vi "Zernike_to_Mirror_Mode_Converter_v01.vi"(2 "Zernike Mode Amplitude":dbl, 3 "Zernike Mode":i32) -> (0 "Mirror Mode Amplitude":dbl[](array[numeric]), 1 "Mirror Modes":i32[](array[numeric]))   [LabVIEW 2015]
uses:
  <vilib>/Utility/file.llb/Read Delimited Spreadsheet (DBL).vi
panel:
  in  "Mirror to Zernike Mode Conversion":path=path "C:/Users/Mlodzianoski/Desktop/Microscope 2 Labview Programs/VIs/DM/MirrorMode_conversion_to_ZernikeMode.txt"
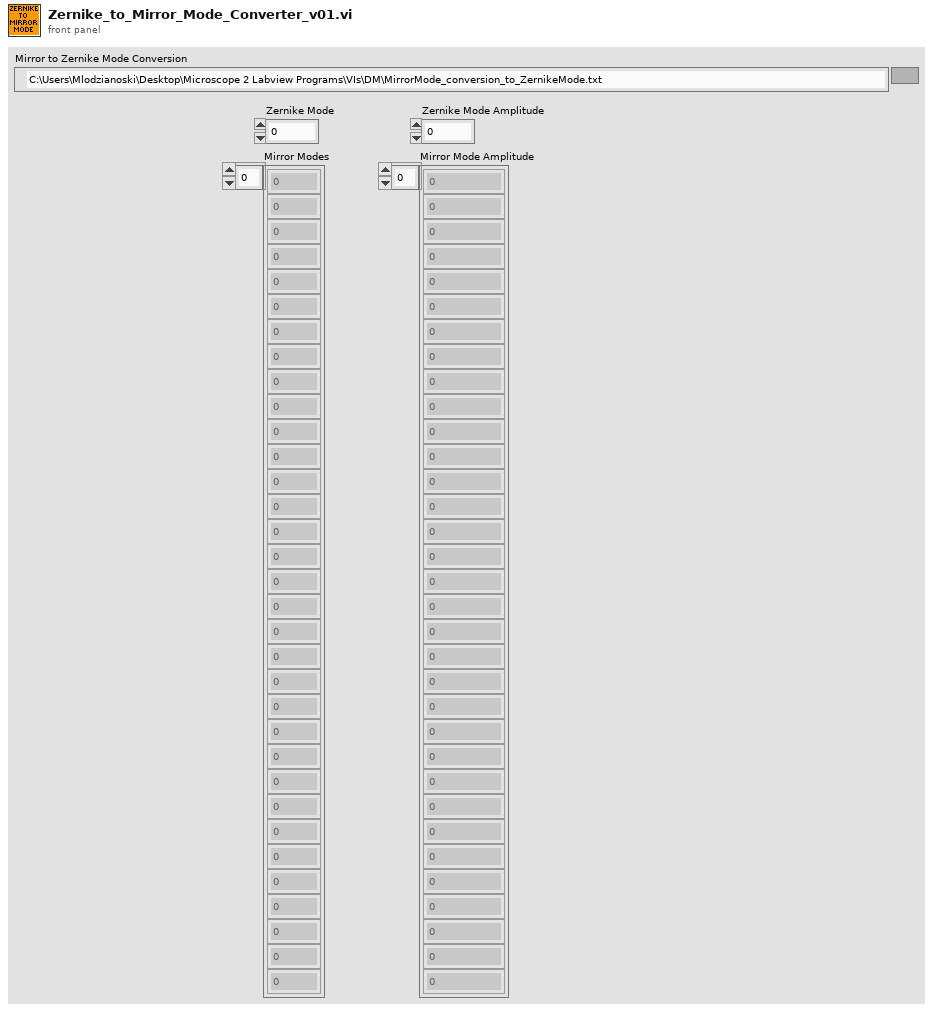
[diagram p1: front panel]
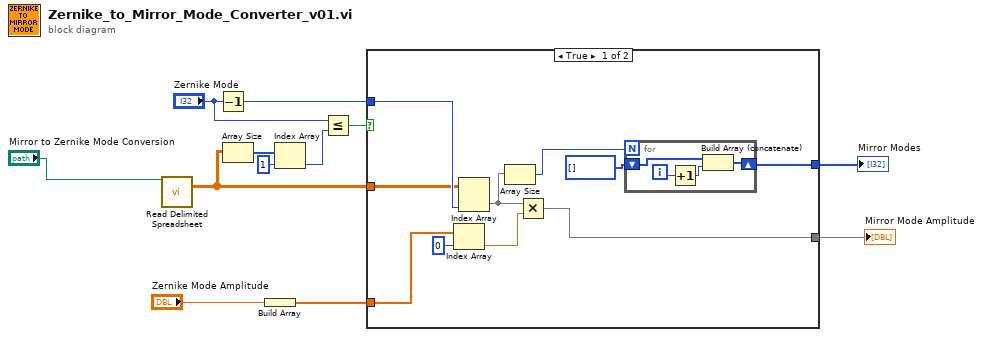
[diagram p0: block diagram]
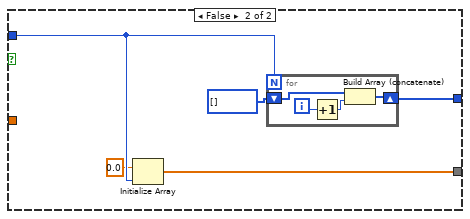
[diagram p2: hidden frame]
diagram:
  n1 = call-poly <vilib>:"Read Delimited Spreadsheet.vi"("file path (dialog if empty)"="Mirror to Zernike Mode Conversion") -> ("all rows"=w7:dbl[][])  [unwired: 9 in, 5 out]
  n2 = Decrement(x="Zernike Mode") -> (x-1=w1:i32)
  n3 = Array Size(array=w7) -> (size(s)=w6:i32[])
  n4 = Build Array("Zernike Mode Amplitude") -> (w9:dbl[])
  n5 = Index Array(array=w6, index=1) -> (element=w4:i32)
  n6 = Less Or Equal?(x="Zernike Mode", y=w4) -> (x <= y?=w3:bool)
  n7 = case shown="True" w3 {
    tunnel: [w22 w31] -> w11
    tunnel: [w21 w27] -> w10
    tunnel: w9 -> [w20 _]
    tunnel: w1 -> [w19 w29]
    tunnel: w7 -> [w13 _]
    frame True {
      n8 = Index Array(array=w20, index=0) -> (element=w14:dbl)
      n9 = Index Array(array=w13, index (col)=w19) -> (element=w16:dbl[])  [unwired: 1 in]
      n10 = Array Size(array=w16) -> (size(s)=w18:i32)
      n11 = Multiply(x=w16, y=w14) -> (x*y=w21:dbl[])
      n12 = for {
        N: w18 -> [_]
        shift-right: [w25] -> w22
        shift-left: i32[] [] -> [w23]
        i -> [w26]
        n13 = Increment(x=w26) -> (x+1=w24:i32)
        n14 = Build Array (concatenate)(w23, w24) -> (w25:i32[])
      }
    }
    frame False {
      n15 = Initialize Array(0.0 ("element"), w29) -> (w27:dbl[])
      n16 = for {
        N: w29 -> [_]
        shift-right: [w34] -> w31
        shift-left: i32[] [] -> [w32]
        i -> [w35]
        n17 = Increment(x=w35) -> (x+1=w33:i32)
        n18 = Build Array (concatenate)(w32, w33) -> (w34:i32[])
      }
    }
  }
  "Mirror Modes" <- w11
  "Mirror Mode Amplitude" <- w10
